vi "Motic Set Exposure.vi"(8 "error in (no error)":errorcluster, 10 "exposure":sgl, 11 "camera":i32) -> (0 "error out":errorcluster, 3 "camera out":i32)   [LabVIEW 2012, in "MoticApi.lvlib"]
doc: "MOTICAPI bool Motic_SetExposure(MUCam_Handle camera, float t);"
uses:
  MoticApi.lvlib
  MoticApi.dll
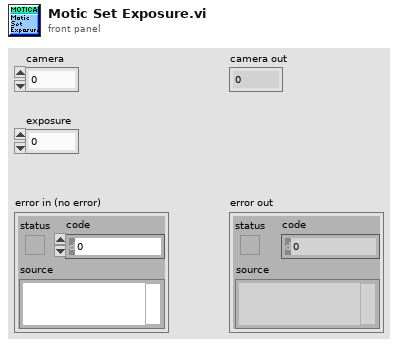
[diagram p1: front panel]
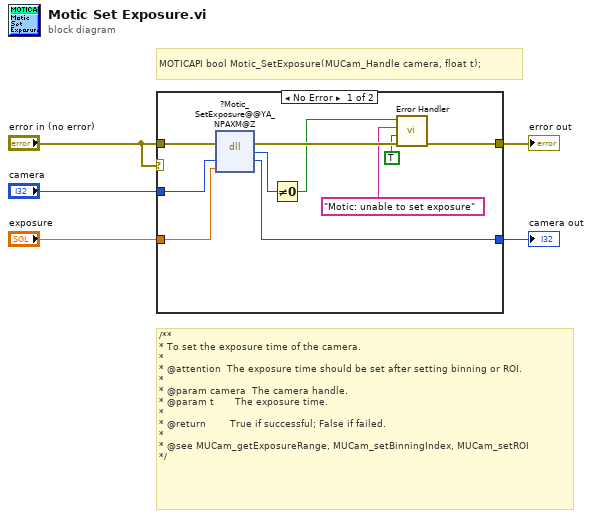
[diagram p0: block diagram]
diagram:
  # "/**\n* To set the exposure time of the camera.\n*\n* @attention  The exposure time should be set after setting binning or ROI.\n*\n* @param camera  The camera handle.\n* @param t       The exposure time.\n*\n* @return        True if successful; False if failed.\n*\n* @see MUCam_getExposureRange, MUCam_setBinningIndex, MUCam_setROI\n*/"
  # "MOTICAPI bool Motic_SetExposure(MUCam_Handle camera, float t);"
  n1 = case shown="No Error" "error in (no error)" {
    tunnel: "camera" -> [w14 w16]
    tunnel: [w13 w16] -> w4
    tunnel: "exposure" -> [w12 _]
    tunnel: "error in (no error)" -> [w11 w17]
    tunnel: [w10 w17] -> w2
    frame No Error {
      n2 = dll-call lib="C:/Users/TTS-Digital/Desktop/MoticApi/MoticApi_git/MoticApi/MoticApi.*" fn="?Motic_SetExposure@@YA_NPAXM@Z"(error in=w11, "camera"=w14, "exposure"=w12) -> (error out=w9:errorcluster, w15:u8, "camera"=w13:i32)  [unwired: 3 in, 1 out]
      n3 = Not Equal To 0?(x=w15) -> (x != 0?=w8:bool)
      n4 = call "Error Handler.vi"("error in (no error)"=w9, "Is warning?"=TRUE, "Error message"="Motic: unable to set exposure", "Function return"=w8) -> ("error out"=w10:errorcluster)  [unwired: 7 in]
    }
    frame Error {
    }
  }
  "camera out" <- w4
  "error out" <- w2
